vi "oax_Generate Simulated Vibration and Tach Signal (Block).vi"(5 "reset?":bool, 7 "fs":dbl=10000.0, 8 "block size [s]":dbl, 9 "order info":T1(array[cluster]) {"envelop config"."low limit" format="%.2f"; "envelop config"."high limit" format="%.2f"; "envelop config"."f" format="%.2f"; "AM selection" items=["None", "Sine", "Triangle"]}, 10 "time period":dbl[](array[numeric]), 11 "speed":dbl[](array[numeric])) -> (2 "Tach Signal":waveform(dbl), 3 "Vibration Signal":waveform(dbl))   [LabVIEW 2017]
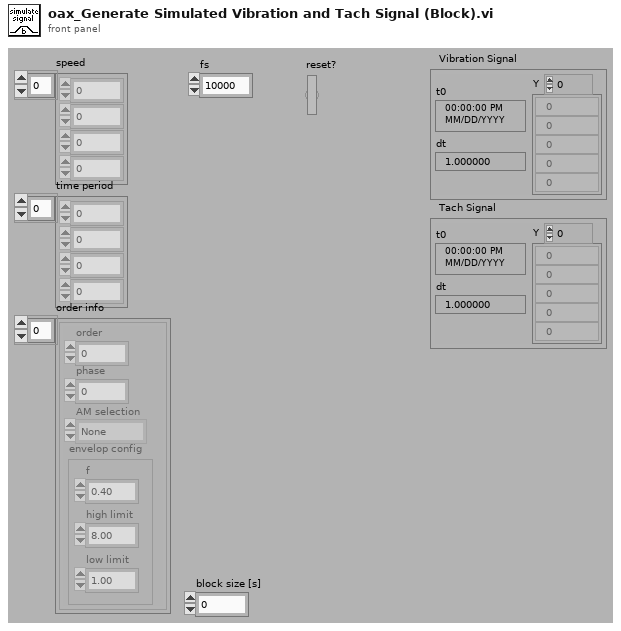
[diagram p1: front panel]
types:
  T1 = cluster{"order":dbl, "phase":dbl, "AM selection":u16, "envelop config":cluster{"f":dbl, "high limit":dbl, "low limit":dbl}}[]
  T2 = cluster{"start/constant speed":dbl, "end speed":dbl, "duration":dbl, "enum":enum16{"Pre period", "Middle period", "Post period"}, "current duration":dbl, "total duration":dbl}[]
  T3 = cluster{"f":dbl, "high limit":dbl, "low limit":dbl}
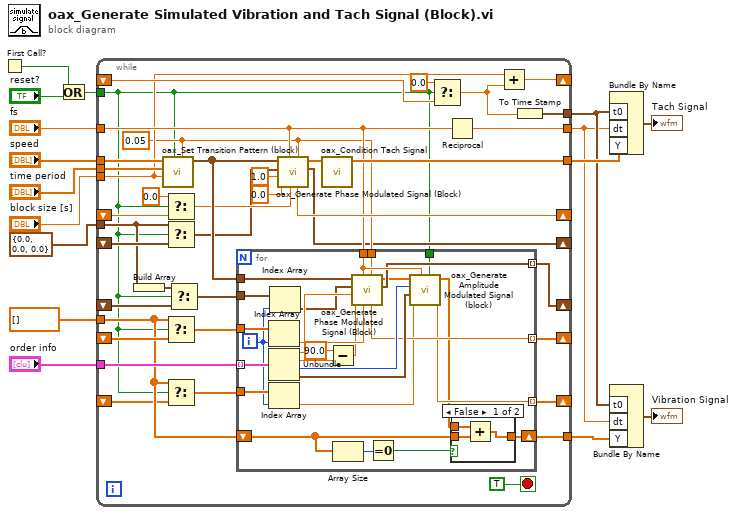
[diagram p0: block diagram]
diagram:
  n1 = First Call?() -> (First Call?: T/F=w8:bool)
  n2 = Or(x=w8, y="reset?") -> (x .or. y?=w6:bool)
  n3 = while {
    tunnel: [w42] -> w16
    tunnel: "order info" -> [w54]
    tunnel: "fs" -> [w38]
    tunnel: "speed" -> [w41]
    tunnel: "time period" -> [w40]
    tunnel: dbl[] [] ("time period 2") -> [w36]
    tunnel: [w44] -> w10
    tunnel: [w37] -> w2
    tunnel: [w53] -> w9
    shift-right: [w51] -> _
    shift-left: _ -> [w49]
    tunnel: w6 -> [w17]
    shift-right: [w47] -> _
    shift-left: _ -> [w46]
    tunnel: "block size [s]" -> [w29]
    shift-right: [w33] -> _
    shift-left: _ -> [w35]
    shift-right: [w28] -> _
    shift-left: _ -> [w31]
    shift-right: [w25] -> _
    shift-left: _ -> [w24]
    tunnel: cluster{"pre":dbl, "mid":dbl, "post":dbl} {"pre"=0.0, "mid"=0.0, "post"=0.0} ("t") -> [w18]
    shift-right: [w22] -> _
    shift-left: _ -> [w21]
    stop <- TRUE stop-if-true
    w27 = 0.05 ("acc transition ratio")
    n4 = Build Array(w18) -> (w19:cluster{"pre":dbl, "mid":dbl, "post":dbl}[])
    n5 = call <vilib>:"oax_Set Transition Pattern (block).vi"("acc transition ratio"=w27, "reset?"=w17, "block size"=w29, "time period"=w40, "speed"=w41) -> ("current speed positions"=w39:T2)  [unwired: 6 in]
    n6 = Select(t=0.0 ("phase"), s=w17, f=w49) -> (s? t:f=w26:dbl)
    n7 = Select(t=w18, s=w17, f=w24) -> (s? t:f=w23:cluster{"pre":dbl, "mid":dbl, "post":dbl})
    n8 = Select(t=w36, s=w17, f=w46) -> (s? t:f=w45:dbl[])
    n9 = Select(t=w36, s=w17, f=w35) -> (s? t:f=w34:dbl[])
    n10 = Select(t=w19, s=w17, f=w21) -> (s? t:f=w20:cluster{"pre":dbl, "mid":dbl, "post":dbl}[])
    n11 = for {
      tunnel: w54 -> [w82] mode=indexing
      tunnel: w38 -> [w76]
      shift-right: [w77] -> w44
      shift-left: w36 -> [w67]
      tunnel: [w75] -> w47 mode=indexing
      tunnel: w45 -> [w74]
      tunnel: w39 -> [w68]
      tunnel: w34 -> [w66]
      tunnel: [w64] -> w33 mode=indexing
      tunnel: w27 -> [w63]
      tunnel: [w62] -> w22 mode=indexing
      tunnel: w20 -> [w60]
      tunnel: w17 -> [w58]
      i -> [w61]
      n12 = Index Array(array=w74, index=w61) -> (element=w73:dbl)
      n13 = Unbundle(w82) -> ("order"=w72:dbl, "phase"=w71:dbl, "AM selection"=w81:u16, "envelop config"=w80:T3)
      n14 = Index Array(array=w66, index=w61) -> (element=w65:dbl)
      n15 = Index Array(array=w60, index=w61) -> (element=w59:cluster{"pre":dbl, "mid":dbl, "post":dbl})
      n16 = Subtract(x=90.0, y=w71) -> (x-y=w69:dbl)
      n17 = Array Size(array=w67) -> (size(s)=w79:i32)
      n18 = call <vilib>:"oax_Generate Phase Modulated Signal (Block).vi"("acc transition ratio"=w63, "init phase"=w73, "fs"=w76, "phase"=w69, "order"=w72, "passed samples in"=w59, "current speed positions"=w68) -> ("passed samples in"=w62:cluster{"pre":dbl, "mid":dbl, "post":dbl}, "y"=w57:dbl[], "final phase"=w75:dbl)  [unwired: 2 in]
      n19 = Equal To 0?(x=w79) -> (x = 0?=w78:bool)
      n20 = call <vilib>:"oax_Generate Amplitude Modulated Signal (block).vi"("reset?"=w58, "fs"=w76, "phase in"=w65, "envelop config"=w80, "AM selection"=w81, "x"=w57) -> ("phase out"=w64:dbl, "AM modulated signal"=w56:dbl[])  [unwired: 4 in]
      n21 = case shown="False" w78 {
        tunnel: w67 -> [w84 _]
        tunnel: [w83 w86] -> w77
        tunnel: w56 -> [w85 w86]
        frame False {
          n22 = Add(x=w85, y=w84) -> (x+y=w83:dbl[])
        }
        frame True {
        }
      }
    }
    n23 = call <vilib>:"oax_Generate Phase Modulated Signal (Block).vi"("acc transition ratio"=w27, "init phase"=w26, "fs"=w38, "phase"=0.0, "order"=1.0, "passed samples in"=w23, "current speed positions"=w39) -> ("passed samples in"=w25:cluster{"pre":dbl, "mid":dbl, "post":dbl}, "y"=w43:dbl[], "final phase"=w51:dbl)  [unwired: 2 in]
    n24 = call <vilib>:"oax_Condition Tach Signal.vi"("tach in"=w43) -> ("tach out"=w42:dbl[])  [unwired: 10 in]
    n25 = Select(t=0.0, s=w17, f=w31) -> (s? t:f=w30:dbl)
    n26 = Reciprocal(x=w38) -> (1/x=w37:dbl)
    n27 = Add(x=w29, y=w30) -> (x+y=w28:dbl)
    n28 = To Time Stamp(1:w30) -> (0:w53:timestamp)
  }
  n29 = Bundle By Name("t0"=w9, "dt"=w2, "Y"=w16) -> (→"Tach Signal":waveform(dbl))  [unwired: 1 in]
  n30 = Bundle By Name("t0"=w9, "dt"=w2, "Y"=w10) -> (→"Vibration Signal":waveform(dbl))  [unwired: 1 in]
